vi "HART_Interpret response.vi"(8 "error in":errorcluster, 11 "byte array":u8[](array[numeric]) format="%.0x") -> (0 "error out":errorcluster, 1 "Data bytes":u8[](array[numeric]) format="%.0x", 2 "Respons on\nCommand":u8 format="%.0x", 3 "Device Address\n(5 bytes)":u8[](array[numeric]) format="%.0x", 4 "Status (2 bytes)":u8[](array[numeric]) format="%.0x")   [LabVIEW 2016]
doc: "Reconstruction of ASCII characters from Packed (6bist ASCII) data format"
panel:
  out "Header\nindex":i32
  out "Calulated Checksum":u8 format="%.0x"
  out "Checksum":u8 format="%.0x"
  out "ByteCount":u8 format="%.0x"
  out "Acknowledge":bool
  out "read Acknowledge":u8 format="%.0x"
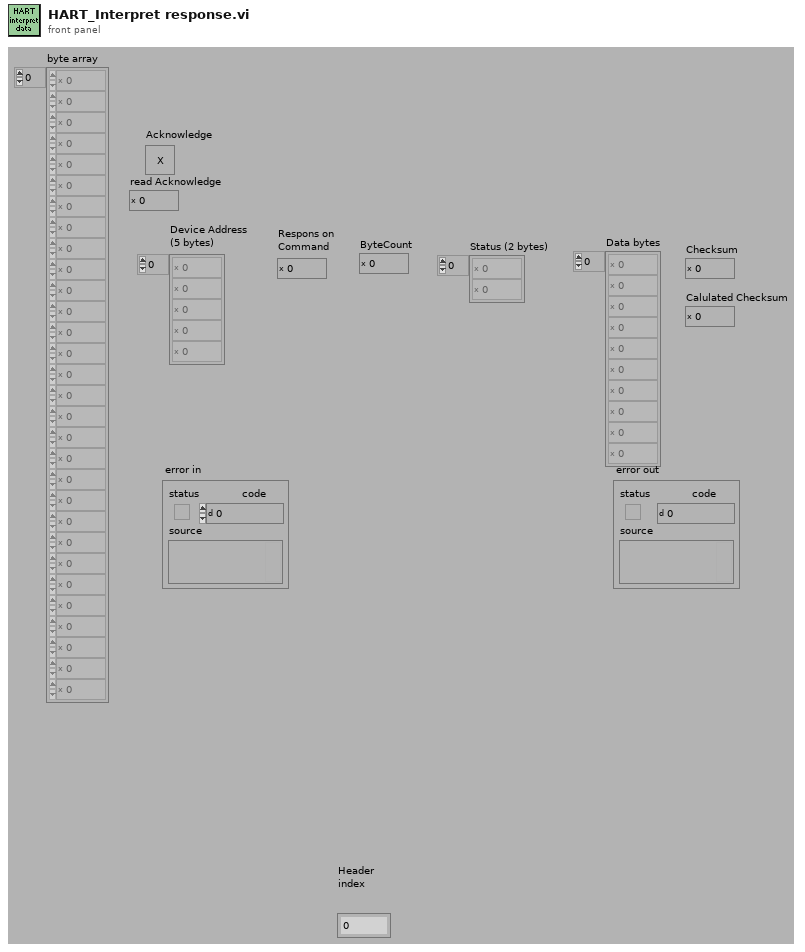
[diagram p1: front panel]
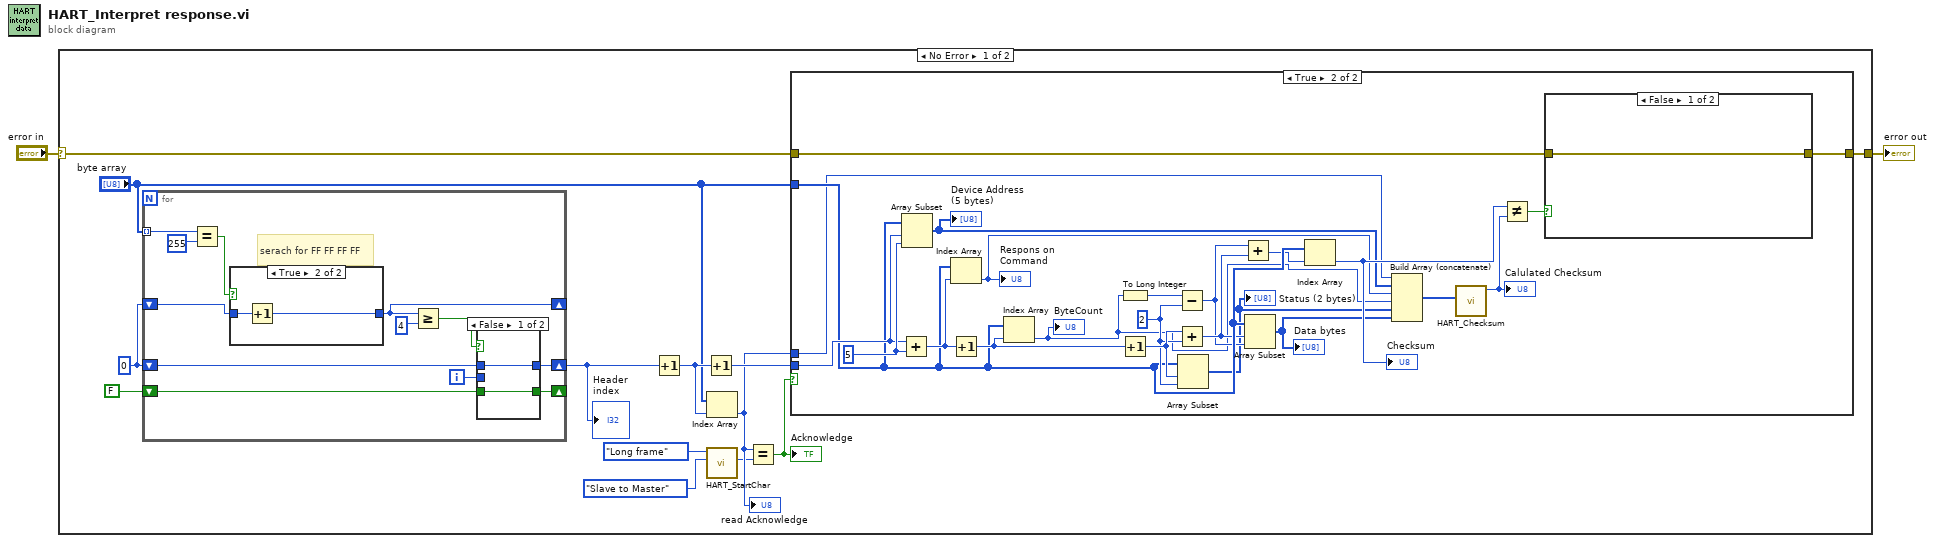
[diagram p0: block diagram]
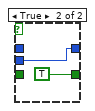
[diagram p2: hidden frame]
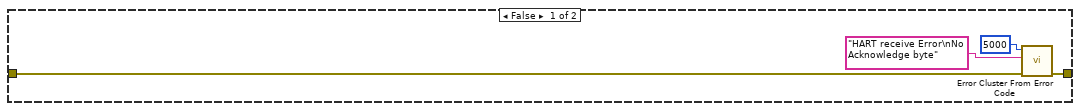
[diagram p4: hidden frame]
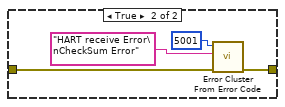
[diagram p5: hidden frame]
diagram:
  n1 = case shown="No Error" "error in" {
    selector: "error in" -> [w9 w66]
    tunnel: [w10 w66] -> w2
    frame No Error {
      w8 = 0
      n2 = for {
        tunnel: "byte array" -> [w27] mode=indexing
        shift-right: [w23] -> _
        shift-left: w8 -> [w26]
        shift-right: [w20] -> w6
        shift-left: w8 -> [w22]
        shift-right: [w17] -> _
        shift-left: FALSE -> [w16]
        i -> [w21]
        # "serach for FF FF FF FF"
        n3 = Equal?(x=w27, y=u8 255 ("element")) -> (x = y?=w19:bool)
        n4 = case shown="True" w19 {
          tunnel: w26 -> [_ w33]
          tunnel: [_ w32] -> w23
          frame False {
          }
          frame True {
            n5 = Increment(x=w33) -> (x+1=w32:i32)
          }
        }
        n6 = Greater Or Equal?(x=w23, y=4) -> (x >= y?=w18:bool)
        n7 = case shown="False" w18 {
          tunnel: w22 -> [w29 _]
          tunnel: w21 -> [_ w31]
          tunnel: [w29 w31] -> w20
          tunnel: [w28 TRUE] -> w17
          tunnel: w16 -> [w28 _]
          frame False {
          }
          frame True {
          }
        }
      }
      "Header\nindex" <- w6
      n8 = Increment(x=w6) -> (x+1=w5:i32)
      n9 = Increment(x=w5) -> (x+1=w13:i32)
      n10 = Index Array(array="byte array", index=w5) -> (element=w12:u8)
      "read Acknowledge" <- w12
      n11 = call "HART_StartChar.vi"("Message type"=enum16{"Master to Slave", "Slave to Master"}."Slave to Master", "Address type"=enum16{"Short frame", "Long frame"}."Long frame") -> ("start character"=w11:u8)  [unwired: 9 in]
      n12 = Equal?(x=w12, y=w11) -> (x = y?=w3:bool)
      "Acknowledge" <- w3
      n13 = case shown="True" w3 {
        tunnel: w13 -> [_ w59]
        tunnel: "byte array" -> [_ w54]
        tunnel: w12 -> [_ w44]
        tunnel: w9 -> [w36 w40]
        tunnel: [w35 w39] -> w10
        frame False {
          n14 = call <vilib>:"Error Cluster From Error Code.vi"("error in (no error)"=w36, "error message (\"\")"="HART receive Error\nNo Acknowledge byte", "error code (0)"=5000) -> ("error out"=w35:errorcluster)  [unwired: 6 in]
        }
        frame True {
          w55 = 2 ("Array Length")
          w60 = 5 ("Array Length")
          n15 = Add(x=w59, y=w60) -> (x+y=w58:i32)
          n16 = Array Subset(array=w54, index=w59, length=w60) -> (w49:u8[])
          "Device Address\n(5 bytes)" <- w49
          n17 = Index Array(array=w54, index=w58) -> (element=w48:u8)
          "Respons on\nCommand" <- w48
          n18 = Increment(x=w58) -> (x+1=w57:i32)
          n19 = Index Array(array=w54, index=w57) -> (element=w47:u8)
          "ByteCount" <- w47
          n20 = To Long Integer(number=w47) -> (32bit integer=w38:i32)
          n21 = Increment(x=w57) -> (x+1=w56:i32)
          n22 = Subtract(x=w38, y=w55) -> (x-y=w51:i32)
          n23 = Add(x=w56, y=w55) -> (x+y=w52:i32)
          n24 = Array Subset(array=w54, index=w56, length=w55) -> (w46:u8[])
          "Status (2 bytes)" <- w46
          n25 = Add(x=w51, y=w52) -> (x+y=w50:i32)
          n26 = Array Subset(array=w54, index=w52, length=w51) -> (w45:u8[])
          "Data bytes" <- w45
          n27 = Index Array(array=w54, index=w50) -> (element=w53:u8)
          "Checksum" <- w53
          n28 = Build Array (concatenate)(w44, w49, w48, w47, w46, w45) -> (w43:u8[])
          n29 = call "HART_Checksum.vi"("message"=w43) -> ("Checksum"=w42:u8)  [unwired: 9 in, 1 out]
          "Calulated Checksum" <- w42
          n30 = Not Equal?(x=w53, y=w42) -> (x != y?=w41:bool)
          n31 = case shown="False" w41 {
            tunnel: w40 -> [w61 w63]
            tunnel: [w61 w62] -> w39
            frame False {
            }
            frame True {
              n32 = call <vilib>:"Error Cluster From Error Code.vi"("error in (no error)"=w63, "error message (\"\")"="HART receive Error\nCheckSum Error", "error code (0)"=5001) -> ("error out"=w62:errorcluster)  [unwired: 6 in]
            }
          }
        }
      }
    }
    frame Error {
    }
  }
  "error out" <- w2
